vi "BD Timestamp to Labview TimeStamp.vi"(1 "BD Time Stamp":string) -> (0 "time stamp":timestamp)   [LabVIEW 2020]
uses:
  <vilib>/Utility/miscctls.llb/LVDateTimeRec.ctl
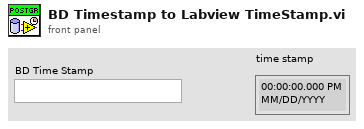
[diagram p1: front panel]
types:
  T1 = typedef "LVDateTimeRec.ctl" = cluster{"fractional second":dbl, "second":i32, "minute":i32, "hour":i32, "day of month":i32, "month":i32, "year":i32, "day of week":i32, "day of year":i32, "DST":i32}
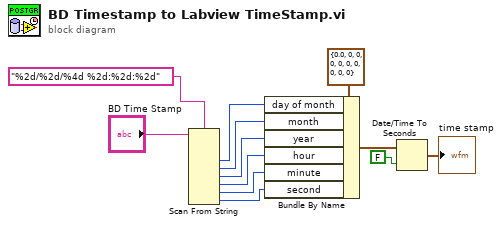
[diagram p0: block diagram]
diagram:
  n1 = Scan From String(format string="%2d/%2d/%4d %2d:%2d:%2d", input string="BD Time Stamp") -> (output 1=w8:i32, output 2=w7:i32, output 3=w6:i32, output 4=w1:i32, output 5=w5:i32, output 6=w4:i32)  [unwired: 8 in, 3 out]
  n2 = Bundle By Name(cluster=T1 {"fractional second"=0.0, "second"=0, "minute"=0, "hour"=0, "day of month"=0, "month"=0, "year"=0, "day of week"=0, "day of year"=0, "DST"=0} ("date time rec"), "day of month"=w8, "month"=w7, "year"=w6, "hour"=w1, "minute"=w5, "second"=w4) -> (w12:T1)
  n3 = Date/Time To Seconds(1:FALSE ("is UTC (F)"), 2:w12) -> (0:→"time stamp":timestamp)
